vi "BGAndSrewImage.vi"(7 "index":i32, 8 "error in (no error)":errorcluster, 9 "BG Image":T1, 10 "Image":T1, 11 "S arrays.S 0":i32[][](array[numeric])) -> (0 "error out":errorcluster, 1 "empty image":bool, 3 "Image Out":T1, 4 "time 2":u32)   [LabVIEW 2020]
uses:
  <vilib>/vision/Image Controls.llb/IMAQ Image.ctl
  <vilib>/vision/NI_Vision_Development_Module.lvlib
panel:
  out "time:filter":u32
  out "time:screw":u32
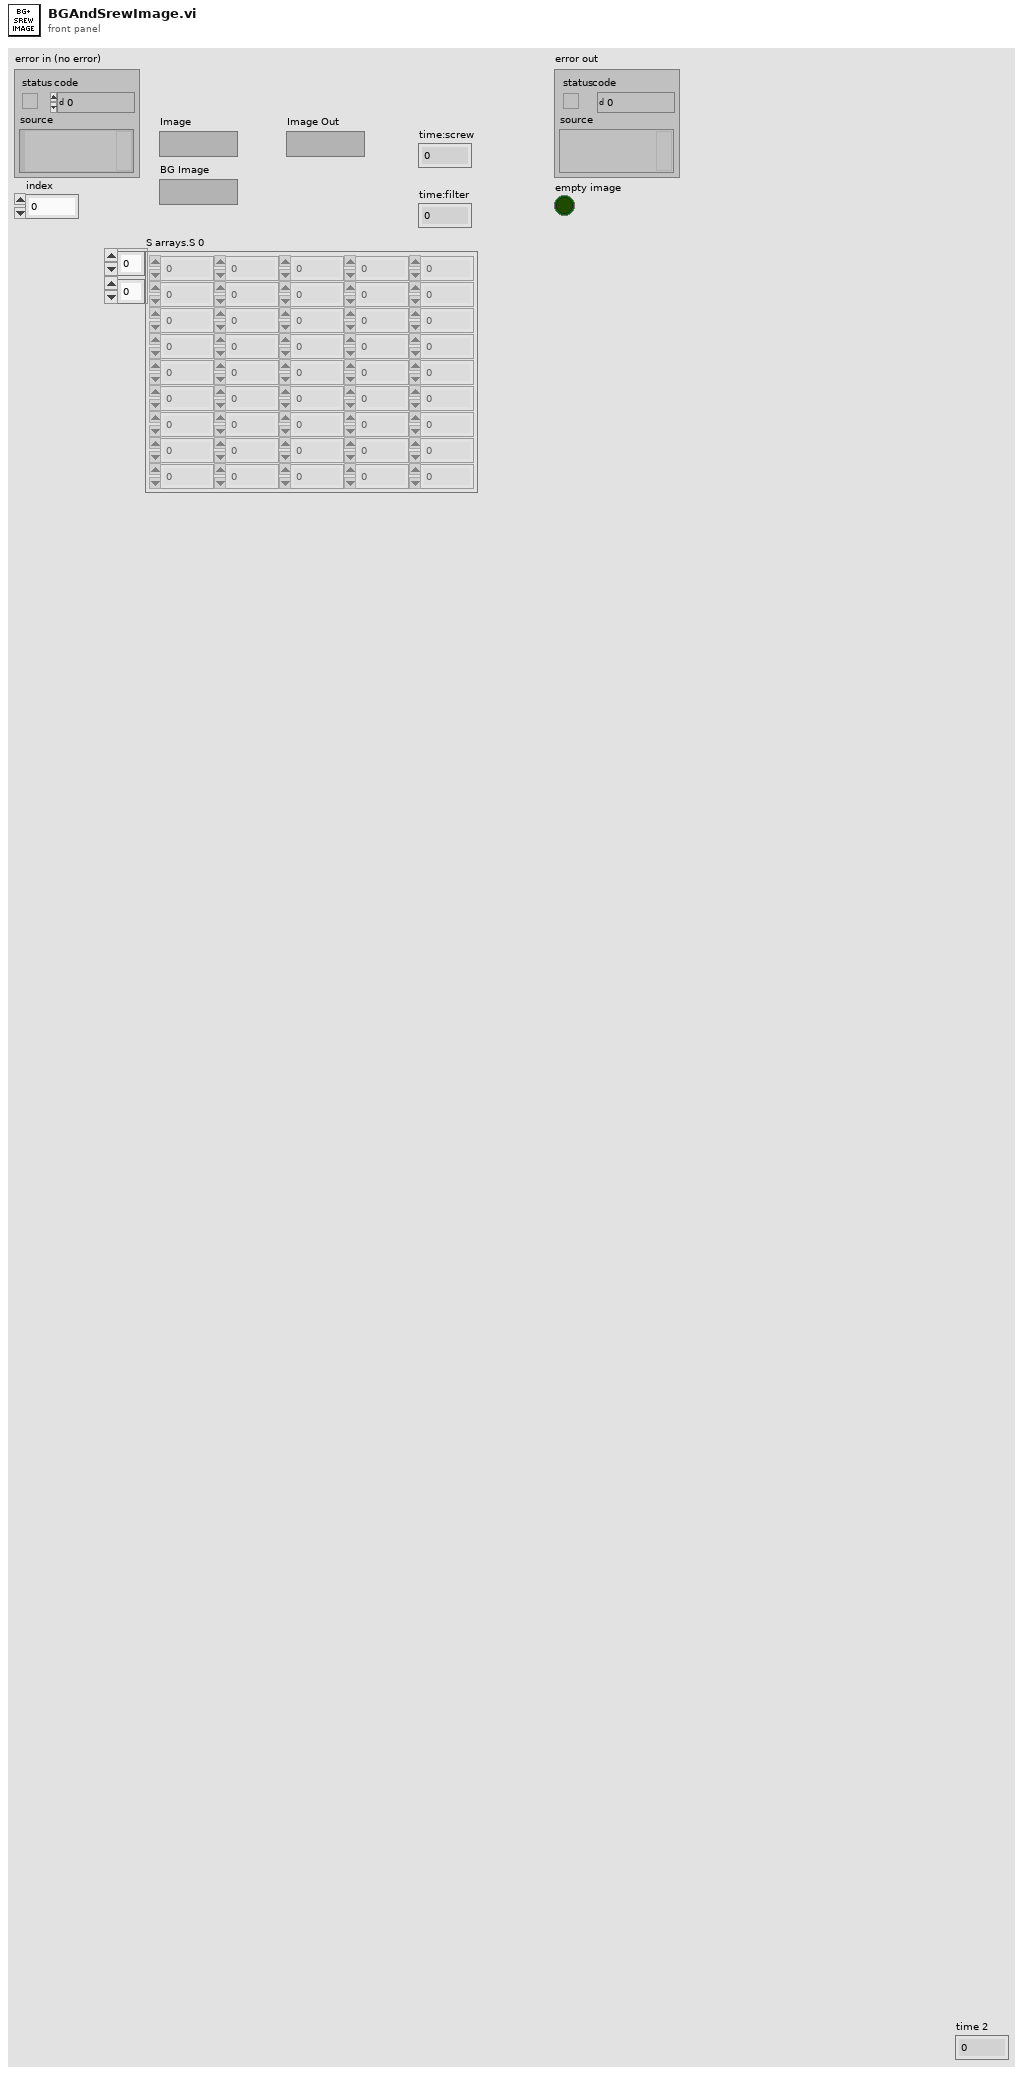
[diagram p1: front panel]
types:
  T1 = typedef "IMAQ Image.ctl" = refnum<image>
  T2 = cluster{"X Size":i32, "Y Size":i32, "Order #":i32}
  T3 = cluster{"X Size":i32, "Y Size":i32, "% Tolerance":i32}
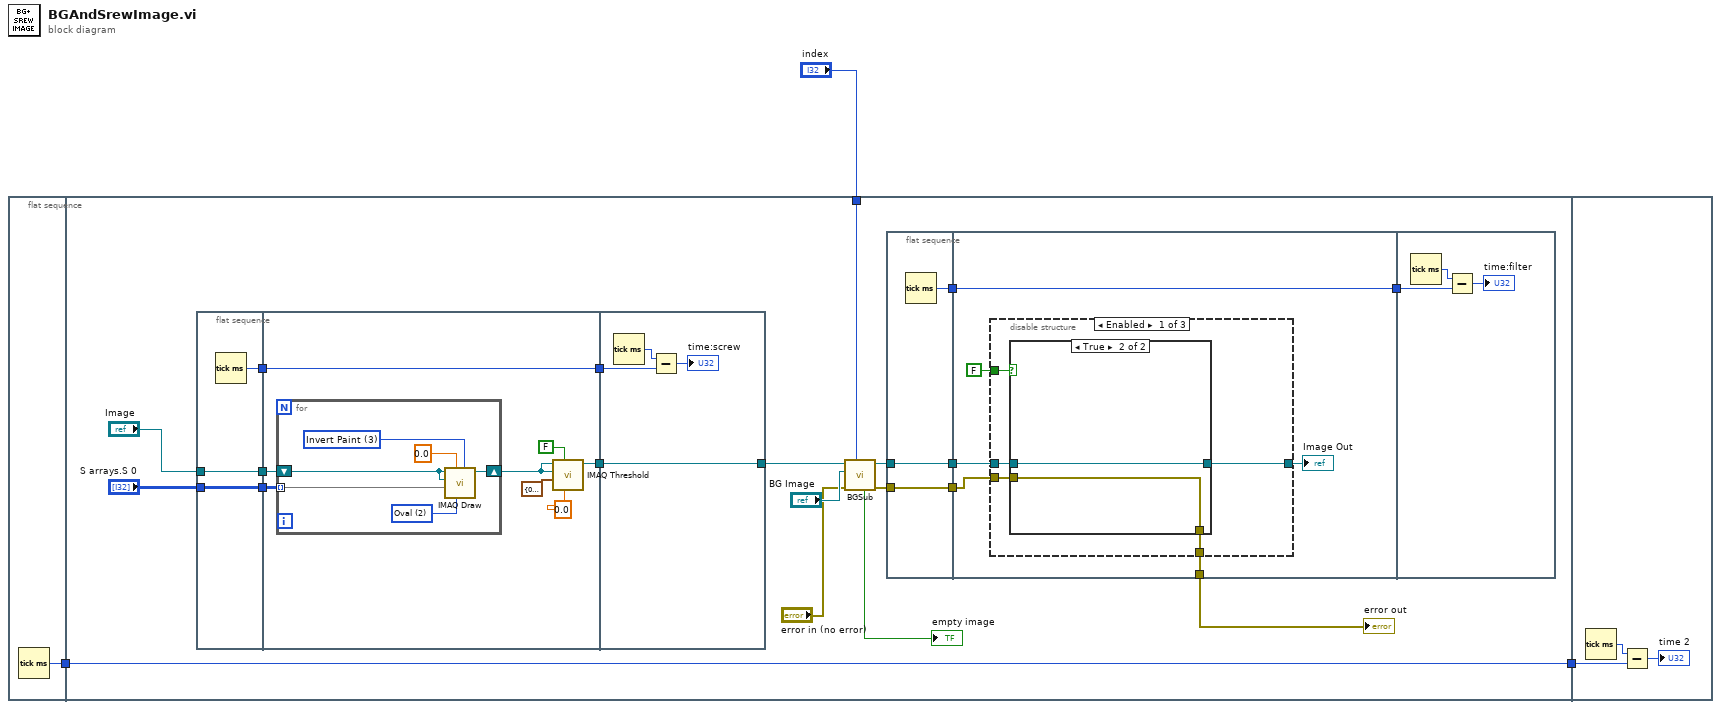
[diagram p0: block diagram]
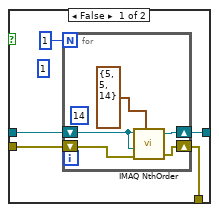
[diagram p2: hidden frame]
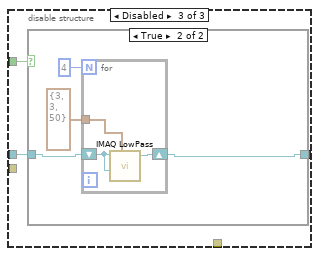
[diagram p4: hidden frame]
diagram:
  n1 = flat-sequence {
    tunnel: [w4] -> w2
    tunnel: [w23] -> w3
    tunnel: w2 -> [w23]
    tunnel: "index" -> [w5]
    tunnel: w3 -> [w87]
    frame #0 {
      n2 = Tick Count (ms)() -> (millisecond timer value=w4:u32)
    }
    frame #1 {
      n3 = flat-sequence {
        tunnel: "Image" -> [w67]
        tunnel: "S arrays.S 0" -> [w68]
        tunnel: [w68] -> w21
        tunnel: [w67] -> w20
        tunnel: [w66] -> w19
        tunnel: [w70] -> w22
        tunnel: w21 -> [w76]
        tunnel: w20 -> [w75]
        tunnel: w19 -> [w69]
        tunnel: [w69] -> w18
        tunnel: [w86] -> w14
        tunnel: w22 -> [w86]
        tunnel: w18 -> [w83]
        frame #0 {
          n4 = Tick Count (ms)() -> (millisecond timer value=w66:u32)
        }
        frame #1 {
          n5 = for {
            shift-right: [w81] -> w71
            shift-left: w75 -> [w82]
            tunnel: w76 -> [w78] mode=indexing
            w80 = u16 2 items=["Line", "Rectangle", "Oval"] ("Shape to draw")
            w79 = u16 3 items=["Frame", "Paint", "Invert Frame", "Invert Paint"] ("Draw Mode")
            n6 = call "IMAQ Draw"("Draw Mode"=w79, "Shape to draw"=w80, "Pixel Color"=sgl 0.0, "Coordinates"=w78, "Image Dst"=w82, "Image Src"=w82) -> ("Image Dst Out"=w81:T1)  [unwired: 4 in, 1 out]
          }
          n7 = call "IMAQ Threshold"("Replace Value"=sgl 0.0, "Keep/Replace Value (Replace)"=FALSE, "Range"=cluster{"Lower value":sgl, "Upper value":sgl} {"Lower value"=0.0, "Upper value"=999999.0}, "Image Dst"=w71, "Image Src"=w71) -> ("Image Dst Out"=w70:T1)  [unwired: 5 in, 1 out]
        }
        frame #2 {
          n8 = Tick Count (ms)() -> (millisecond timer value=w84:u32)
          n9 = Subtract(x=w84, y=w83) -> (x-y=→"time:screw":u32)
        }
      }
      n10 = call "BGSub.vi"("index"=w5, "error in (no error)"="error in (no error)", "BG IN"="BG Image", "raw Image In"=w14) -> ("error out"=w7:errorcluster, "Refnum out"=w13:T1, "empty image"=→"empty image":bool)  [unwired: 5 in]
      n11 = flat-sequence {
        tunnel: w13 -> [w27]
        tunnel: [w27] -> w17
        tunnel: [w26] -> w15
        tunnel: [w25] -> w8
        tunnel: w7 -> [w25]
        tunnel: w17 -> [w31]
        tunnel: [w33] -> w16
        tunnel: w15 -> [w33]
        tunnel: w8 -> [w29]
        tunnel: [w28] -> w6
        tunnel: w16 -> [w63]
        frame #0 {
          n12 = Tick Count (ms)() -> (millisecond timer value=w26:u32)
        }
        frame #1 {
          n13 = disable-structure shown="Enabled" {
            disable-tunnel: [w37 w51 w53] -> w32
            disable-tunnel: w31 -> [w38 w51 w54]
            disable-tunnel: FALSE ("empty array") -> [w36 _ w52]
            disable-tunnel: w29 -> [w35 _ _]
            disable-tunnel: [w34 _ _] -> w28
            frame Enabled {
              n14 = case shown="True" w36 {
                tunnel: w38 -> [w43 w50]
                tunnel: [w42 w50] -> w37
                tunnel: w35 -> [w40 w49]
                tunnel: [w39 w49] -> w34
                frame False {
                  (unwired) 1
                  n15 = for {
                    N: 1 -> [_]
                    shift-right: [w46] -> w42
                    shift-left: w43 -> [w48]
                    shift-right: [w44] -> w39
                    shift-left: w40 -> [w45]
                    (unwired) 14 ("Order #")
                    n16 = call "IMAQ NthOrder"("Image Src"=w48, "Size & Order #"=T2 {"X Size"=5, "Y Size"=5, "Order #"=14}, "Image Dst"=w48, "error in (no error)"=w45) -> ("Image Dst Out"=w46:T1, "error out"=w44:errorcluster)  [unwired: 3 in]
                  }
                }
                frame True {
                }
              }
            }
            frame Disabled {
            }
            frame Disabled {
              n17 = case shown="True" w52 {
                tunnel: w54 -> [w55 w56]
                tunnel: [w55 w57] -> w53
                frame False {
                }
                frame True {
                  n18 = for {
                    N: 4 -> [_]
                    tunnel: T3 {"X Size"=3, "Y Size"=3, "% Tolerance"=50} ("Size & Tolerance") -> [w61]
                    shift-right: [w60] -> w57
                    shift-left: w56 -> [w62]
                    n19 = call "IMAQ LowPass"("Image Src"=w62, "Size & Tolerance"=w61, "Image Dst"=w62) -> ("Image Dst Out"=w60:T1)  [unwired: 4 in, 1 out]
                  }
                }
              }
            }
          }
          "Image Out" <- w32
        }
        frame #2 {
          n20 = Tick Count (ms)() -> (millisecond timer value=w65:u32)
          n21 = Subtract(x=w65, y=w63) -> (x-y=→"time:filter":u32)
        }
      }
      "error out" <- w6
    }
    frame #2 {
      n22 = Tick Count (ms)() -> (millisecond timer value=w88:u32)
      n23 = Subtract(x=w88, y=w87) -> (x-y=→"time 2":u32)
    }
  }
